vi "Event Messenger Channel Lesson 3.vi"() -> ()   [LabVIEW 2019]
doc: "Lesson 3 shows how multiple producers can trigger the same event, including the consumer producing events for itself. It also demonstrates that any loop can be used to stop all of the loops."
uses:
  <extravilib>/ChannelInstances/Event Messenger-str/Instantiate.vi
  <extravilib>/ChannelInstances/Event Messenger-str/))Channel.vi
  <extravilib>/ChannelInstances/Event Messenger-str.lvlib
panel:
  in  "Stop Consumer":bool
  out "Command Received":string
  in  "Stop Beta":bool
  in  "Stop Alpha":bool
  # "Overview: This VI demonstrates how to use the Event Messenger channel wire.\n\nLesson 3 shows how multiple producers can trigger the same event, including the consumer producing events for itself. It also demonstrates that any loop can be used to stop all of the loops.\n\nInstructions:\n1. Run the VI. Notice that both Producers run at the same rate. The consumer in this lesson runs as fast as it can, so in this example, stopping should be pretty close to immediate because events do not get backlogged.\n2. Stop the VI by hitting any of the STOP or ABORT buttons. Each button is part of a separate loop, but because of the communication provided by the channel wire, a stop signal raised by any of the loops will stop all of the loops. The STOP will do a lazy stop, allowing remaining elements to be processed. ABORT will stop immediately.\n3. Open the block diagram. Review the comments there to see how this VI works."
  # "Producer Alpha"
  # "Producer Beta"
  # "Consumer"
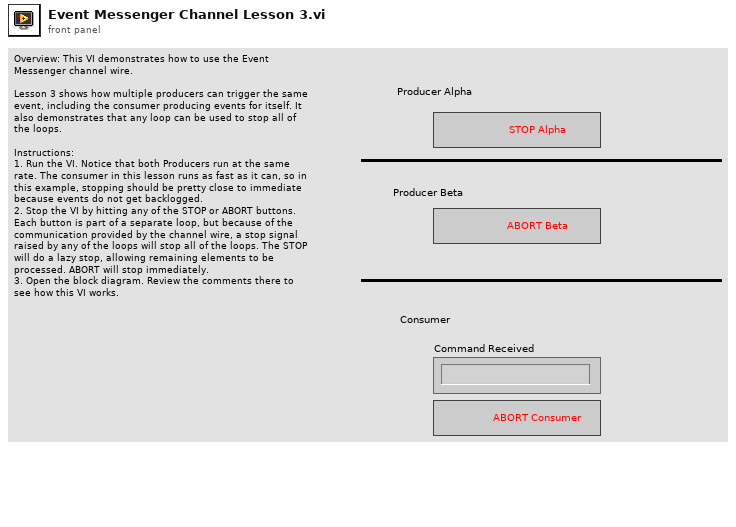
[diagram p1: front panel]
types:
  T1 = typedef "Event Messenger-str.lvlib/))Channel.ctl" = refnum<queue>
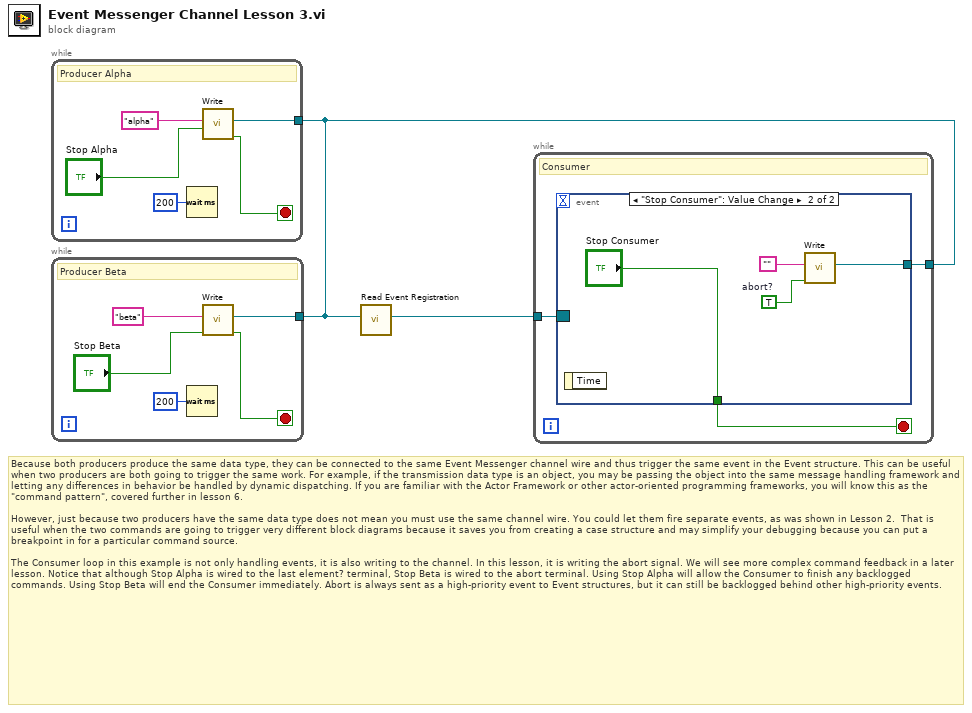
[diagram p0: block diagram]
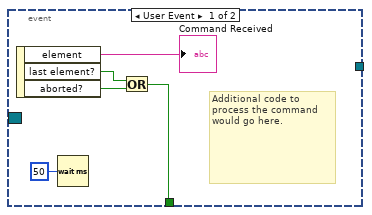
[diagram p2: hidden frame]
diagram:
  # "Because both producers produce the same data type, they can be connected to the same Event Messenger channel wire and thus trigger the same event in the Event structure. This can be useful when two producers are both going to trigger the same work. For example, if the transmission data type is an object, you may be passing the object into the same message handling framework and letting any differences in behavior be handled by dynamic dispatching. If you are familiar with the Actor Framework or other actor-oriented programming frameworks, you will know this as the \"command pattern\", covered further in lesson 6.\n\nHowever, just because two producers have the same data type does not mean you must use the same channel wire. You could let them fire separate events, as was shown in Lesson 2.  That is useful when the two commands are going to trigger very different block diagrams because it saves you from creating a case structure and may simplify your debugging because you can put a breakpoint in for a particular command source.\n\nThe Consumer loop in this example is not only handling events, it is also writing to the channel. In this lesson, it is writing the abort signal. We will see more complex command feedback in a later lesson. Notice that although Stop Alpha is wired to the last element? terminal, Stop Beta is wired to the abort terminal. Using Stop Alpha will allow the Consumer to finish any backlogged commands. Using Stop Beta will end the Consumer immediately. Abort is always sent as a high-priority event to Event structures, but it can still be backlogged behind other high-priority events."
  n1 = while {
    tunnel: [w7] -> w2
    stop <- w5 stop-if-true
    # "Producer Alpha"
    n2 = Wait (ms)(milliseconds to wait=u32 200) -> ()  [unwired: 1 out]
    n3 = call <extravilib>:"Write.vi"("last element? (F)"="Stop Alpha", "element"="alpha") -> ("done?"=w5:bool, "channel"=w7:T1)  [unwired: 8 in]
  }
  n4 = while {
    tunnel: w2 -> [w10]
    stop <- w12 stop-if-true
    # "Producer Beta"
    n5 = Wait (ms)(milliseconds to wait=u32 200) -> ()  [unwired: 1 out]
    n6 = call <extravilib>:"Write.vi"("abort (F)"="Stop Beta", "element"="beta") -> ("done?"=w12:bool, "channel"=w10:T1)  [unwired: 8 in]
  }
  n7 = call <extravilib>:"Read Event Registration.vi"("channel"=w2) -> ("event registration refnum"=w1:refnum<event-registration>)  [unwired: 10 in]
  n8 = while {
    tunnel: w1 -> [w14]
    tunnel: w2 -> [w13]
    stop <- w15 stop-if-true
    # "Consumer"
    n9 = event shown="[1] \"Stop Consumer\": Value Change" {
      selector: w14 -> [_ _]
      dyn-events: _ -> [_ _]
      timeout: _ -> [_ _]
      tunnel: [w16 "Stop Consumer"] -> w15
      tunnel: [_ w21] -> w13
      event User Event {
        # "Additional code to process the command would go here."
        n10 = event-data() -> ("element"=→"Command Received":string, "last element?"=w17:bool, "aborted?"=w18:bool)  [unwired: 1 in]
        n11 = Wait (ms)(milliseconds to wait=u32 50) -> ()  [unwired: 1 out]
        n12 = Or(x=w17, y=w18) -> (x .or. y?=w16:bool)
      }
      event "Stop Consumer": Value Change {
        w23 = TRUE  # abort?
        n13 = event-data() -> ()  [unwired: 1 in, 1 out]
        n14 = call <extravilib>:"Write.vi"("abort (F)"=w23, "element"="") -> ("channel"=w21:T1)  [unwired: 8 in, 1 out]
      }
    }
  }
